vi "AdaptToInputs.vi"(0 "XRef":T9, 1 "Term Types":T6, 2 "State In":T1) -> (14 "Reply":T4, 16 "State Out":T1)   [LabVIEW 2015, in "Async-And-Forget.xnode"]
uses:
  Async-And-Forget.xnode
  <vilib>/XNodeSupport/XNodeXNodeRef.ctl
  <vilib>/XNodeSupport/XNodeTermTypeIDPairs.ctl
  <vilib>/XNodeSupport/XNodeTermTypeIDPair.ctl
  <vilib>/XNodeSupport/XNodeType.ctl
  <vilib>/XNodeSupport/XNodeString.ctl
  State.ctl
  <vilib>/Utility/miscctls.llb/LVRectTypeDef.ctl
  <vilib>/picture/picture.llb/imagedata.ctl
  <vilib>/XNodeSupport/XNodeStringArray.ctl
  <vilib>/XNodeSupport/NI_XNodeSupport.lvlib
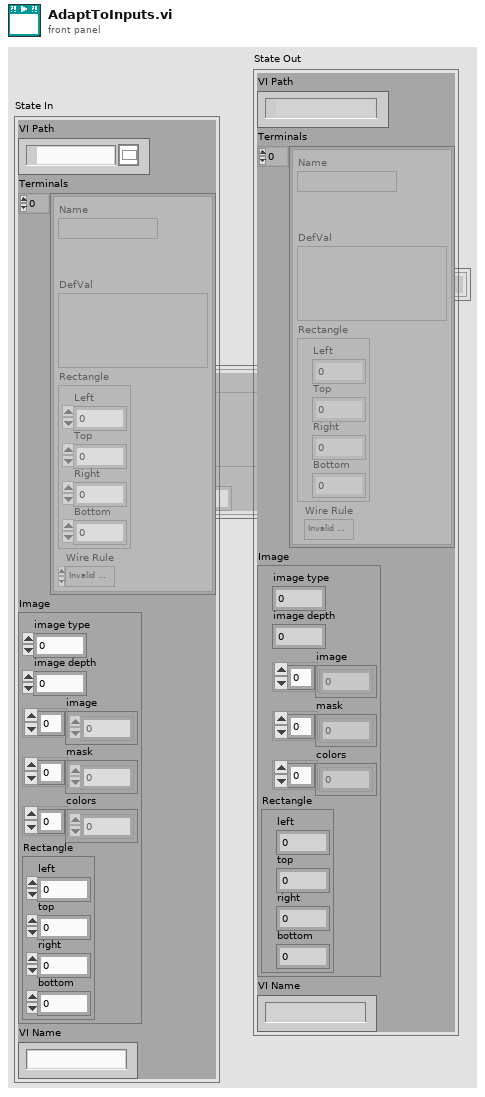
[diagram p1: front panel]
types:
  T1 = typedef "Async-And-Forget.xnode/State.ctl" = cluster{"VI Path":path, "Terminals":cluster{"Name":string, "DefVal":variant, "Rectangle":T2, "Wire Rule":enum16{"Invalid Wire Rule", "Required", "Recommended", "Optional", "Dynamic Dispatch"}}[], "Image":T3, "VI Name":string}
  T2 = typedef "LVRectTypeDef.ctl" = cluster{"Left":i16, "Top":i16, "Right":i16, "Bottom":i16}
  T3 = typedef "imagedata.ctl" = cluster{"image type":i32, "image depth":i32, "image":u8[], "mask":u8[], "colors":u32[], "Rectangle":cluster{"left":i16, "top":i16, "right":i16, "bottom":i16}}
  T4 = typedef "NI_XNodeSupport.lvlib/XNodeStringArray.ctl" = T5[]
  T5 = typedef "NI_XNodeSupport.lvlib/XNodeString.ctl" = string
  T6 = typedef "NI_XNodeSupport.lvlib/XNodeTermTypeIDPairs.ctl" = T7[]
  T7 = typedef "NI_XNodeSupport.lvlib/XNodeTermTypeIDPair.ctl" = cluster{"Type":T8, "Id":T5}
  T8 = typedef "NI_XNodeSupport.lvlib/XNodeType.ctl" = variant
  T9 = typedef "NI_XNodeSupport.lvlib/XNodeXNodeRef.ctl" = refnum<vi>
  T10 = enum16{"Invalid Wire Rule", "Required", "Recommended", "Optional", "Dynamic Dispatch"}[]
  T11 = cluster{"Name":string, "DefVal":variant, "Rectangle":T2, "Wire Rule":enum16{"Invalid Wire Rule", "Required", "Recommended", "Optional", "Dynamic Dispatch"}}[]
  T12 = cluster{"Label.Text":string, "DefVal":variant, "Rectangle":T2, "Wire Rule":enum16{"Invalid Wire Rule", "Required", "Recommended", "Optional", "Dynamic Dispatch"}}[]
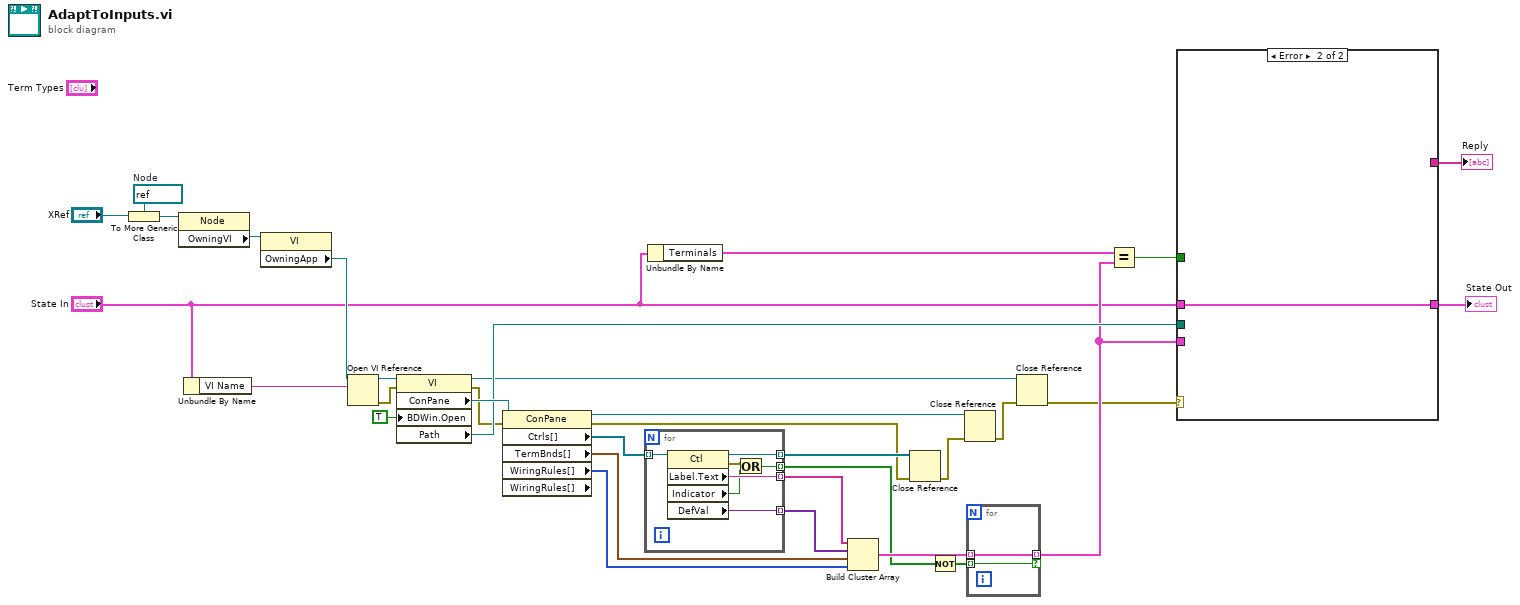
[diagram p0: block diagram]
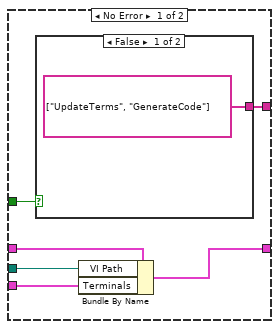
[diagram p2: hidden frame]
diagram:
  w29 = refnum<vi> refnum  # Node
  n1 = To More Generic Class(target class=w29, reference="XRef") -> (generic class reference=w28:refnum<vi>)
  n2 = property class="Node"(reference=w28) -> ("OwningVI"=w27:refnum<vi>)  [unwired: 1 in, 2 out]
  n3 = Unbundle By Name("State In") -> ("VI Name"=w31:string)
  n4 = property class="VI"(reference=w27) -> ("OwningApp"=w26:refnum<vi>)  [unwired: 1 in, 2 out]
  n5 = Open VI Reference(application reference (local)=w26, vi path=w31) -> (vi reference=w33:refnum<vi>, error out=w32:errorcluster)  [unwired: 4 in]
  n6 = property class="VI"(reference=w33, error in=w32, "BDWin.Open"=TRUE ("Block Diagram Window:Open")) -> (reference out=w5:refnum<vi>, error out=w4:errorcluster, "ConPane"=w15:refnum<vi>, "Path"=w14:path)
  n7 = property class="ConPane" props=["Ctrls[]", "TermBnds[]", "WiringRules[]", "WiringRules[]"](reference=w15, error in=w4) -> (reference out=w3:refnum<vi>, error out=w2:errorcluster, "Ctrls[]"=w25:refnum<vi>[], "TermBnds[]"=w23:T2[], "WiringRules[]"=w24:T10)  [unwired: 1 out]
  n8 = for {
    tunnel: w25 -> [w40] mode=indexing
    tunnel: [w39] -> w21 mode=indexing
    tunnel: [w38] -> w22 mode=indexing
    tunnel: [w37] -> w20 mode=indexing
    tunnel: [w34] -> w17 mode=indexing
    n9 = property class="Ctl"(reference=w40) -> (reference out=w37:refnum<vi>, error out=w36:errorcluster, "Label.Text"=w39:string, "Indicator"=w35:bool, "DefVal"=w38:variant)  [unwired: 1 in]
    n10 = Or(x=w36, y=w35) -> (x .or. y?=w34:bool)
  }
  n11 = Unbundle By Name("State In") -> ("Terminals"=w13:T11)
  n12 = Build Cluster Array(w21, w22, w23, w24) -> (w18:T12)
  n13 = Close Reference(reference=w20, error in (no error)=w2) -> (error out=w19:errorcluster)
  n14 = Not(x=w17) -> (.not. x?=w16:bool[])
  n15 = Close Reference(reference=w3, error in (no error)=w19) -> (error out=w6:errorcluster)
  n16 = for {
    tunnel: w18 -> [w42] mode=indexing
    tunnel: [w42] -> w11 mode=indexing if=w41
    tunnel: w16 -> [w41] mode=indexing
  }
  n17 = Close Reference(reference=w5, error in (no error)=w6) -> (error out=w1:errorcluster)
  n18 = Equal?(x=w13, y=w11) -> (x = y?=w12:bool)
  n19 = case shown="Error" w1 {
    tunnel: w14 -> [w48 _]
    tunnel: w12 -> [w47 _]
    tunnel: w11 -> [w46 _]
    tunnel: "State In" -> [w45 w50]
    tunnel: [w44 w50] -> w8
    tunnel: [w43 _] -> w7
    frame No Error {
      n20 = case shown="False" w47 {
        tunnel: [string[] ["UpdateTerms", "GenerateCode"] ("Reply") _] -> w43
        frame False {
        }
        frame True {
        }
      }
      n21 = Bundle By Name(cluster=w45, "VI Path"=w48, "Terminals"=w46) -> (w44:T1)
    }
    frame Error {
    }
  }
  "Reply" <- w7
  "State Out" <- w8
